vi "Structure Handler.vi"() -> ()   [LabVIEW 2010]
uses:
  <vilib>/Utility/miscctls.llb/LV3DPointTypeDef.ctl
  <vilib>/Analysis/Matrix/Datatypes/RealMatrix.ctl
  <vilib>/addons/database/_DB Variant To Data/Database Variant To Data.xnode
  <vilib>/addons/database/Connection.llb/DB Tools Open Connec (Path).vi
  <vilib>/addons/database/Connection.llb/Conn Execute.vi
  <vilib>/addons/database/Recordset.llb/Rec Fetch Recordset Data (R).vi
  <vilib>/addons/database/Recordset.llb/Rec Destroy - Connection.vi
  <vilib>/Analysis/_algsub.llb/Real Vector Norm.vi
  <vilib>/Utility/file.llb/Read From Spreadsheet File (string).vi
  <vilib>/Utility/file.llb/Write To Spreadsheet File (string).vi
  <vilib>/Analysis/baseanly.llb/Real Dot Product.vi
  <vilib>/addons/database/NI_Database_API.lvlib
  <vilib>/picture/3D Picture Control/NI_3D Picture Control.lvlib
  <vilib>/Analysis/NI_AALPro.lvlib
  <vilib>/Analysis/NI_AALBase.lvlib
  <vilib>/Analysis/Matrix/NI_Matrix.lvlib
panel:
  out "Last Structures":T1(array[cluster])
  out "x-y":u32[](array[numeric])
  out "Last Path":path caption="selected path"
  out "PickPoint":T2
  out "GB Subcrystal":T3={"Structure Name"="Batch6_3+111 Quasi-Bulk", "Lattice vector a"=[9.1641, 0.0, 0.0], "Lattice vector b"=[0.0, 7.93635, 0.0], "Lattice vector c"=[0.0, 0.0, 53.7091], "Atoms Array"=[{"Atom Name"="", "Positions (Direct)"=[[0.036896, 0.129554, 0.035254], [0.536896, 0.129554, 0.035254], [0.286896, 0.629554, 0.035254], [0.786896, 0.629554, 0.035254], [0.285415, 0.295133, 0.107673], [0.785415, 0.295133, 0.107673], [0.035415, 0.795133, 0.107673], [0.535415, 0.795133, 0.107673], [0.033615, 0.463308, 0.180101], [0.533615, 0.463308, 0.180101], [0.283615, 0.963308, 0.180101], [0.783615, 0.963308, 0.180101], [0.030844, 0.131453, 0.252535], [0.530844, 0.131453, 0.252535], [0.280844, 0.631453, 0.252535], [0.780844, 0.631453, 0.252535], [0.278379, 0.302058, 0.324923], [0.778379, 0.302058, 0.324923], [0.028379, 0.802058, 0.324923], [0.528379, 0.802058, 0.324923], [0.031198, 0.471844, 0.397363], [0.531198, 0.471844, 0.397363], [0.281198, 0.971844, 0.397363], [0.781198, 0.971844, 0.397363], [0.03247, 0.140643, 0.469814], [0.53247, 0.140643, 0.469814], [0.28247, 0.640643, 0.469814], [0.78247, 0.640643, 0.469814], [0.284308, 0.303948, 0.542263], [0.784308, 0.303948, 0.542263], [0.034308, 0.803948, 0.542263], [0.534308, 0.803948, 0.542263], [0.035944, 0.468219, 0.614701], [0.535944, 0.468219, 0.614701], [0.285944, 0.968219, 0.614701], [0.785944, 0.968219, 0.614701], [0.037813, 0.131858, 0.687216], [0.537813, 0.131858, 0.687216], [0.787813, 0.631858, 0.687216], [0.287813, 0.631858, 0.687216], [0.038238, 0.463759, 0.759817], [0.538238, 0.463759, 0.759817], [0.288238, 0.963758, 0.759817], [0.788238, 0.963758, 0.759817], [0.038639, 0.130134, 0.831025], [0.538639, 0.130134, 0.831025], [0.288639, 0.630134, 0.831025], [0.788639, 0.630134, 0.831025], [0.285712, 0.295024, 0.89873], [0.785712, 0.295024, 0.89873], [0.035712, 0.795024, 0.89873], [0.535712, 0.795024, 0.89873], [0.032596, 0.464879, 0.966384], [0.532596, 0.464879, 0.966384], [0.282596, 0.964879, 0.966384], [0.782596, 0.964879, 0.966384]], "Positions (Cartesian)"=[[0.33811863359999994, 1.0281858879, 1.8934606114], [4.9201686336, 1.0281858879, 1.8934606114], [2.6291436335999996, 4.9963608879, 1.8934606114], [7.2111936336, 4.9963608879, 1.8934606114], [2.6155716014999997, 2.34227878455, 5.7830199243000004], [7.197621601499999, 2.34227878455, 5.7830199243000004], [0.3245466015, 6.31045378455, 5.7830199243000004], [4.9065966014999995, 6.31045378455, 5.7830199243000004], [0.30805122149999997, 3.6769744458, 9.673062619100001], [4.890101221499999, 3.6769744458, 9.673062619100001], [2.5990762215, 7.6451494458, 9.673062619100001], [7.1811262215, 7.6451494458, 9.673062619100001], [0.2826575004, 1.04325701655, 13.5634275685], [4.8647075004, 1.04325701655, 13.5634275685], [2.5736825004, 5.011432016550001, 13.5634275685], [7.155732500399999, 5.011432016550001, 13.5634275685], [2.5510929938999998, 2.3972380083, 17.4513218993], [7.1331429939, 2.3972380083, 17.4513218993], [0.2600679939, 6.3654130083, 17.4513218993], [4.8421179939000005, 6.3654130083, 17.4513218993], [0.28590159179999997, 3.7447191294, 21.3420091033], [4.867951591799999, 3.7447191294, 21.3420091033], [2.5769265918, 7.7128941294, 21.3420091033], [7.158976591799999, 7.7128941294, 21.3420091033], [0.29755832699999996, 1.11619207305, 25.2332871074], [4.879608327, 1.11619207305, 25.2332871074], [2.588583327, 5.08436707305, 25.2332871074], [7.170633327, 5.08436707305, 25.2332871074], [2.6054269428, 2.4122377098, 29.124457693300002], [7.1874769428, 2.4122377098, 29.124457693300002], [0.31440194279999994, 6.3804127098, 29.124457693300002], [4.8964519428, 6.3804127098, 29.124457693300002], [0.32939441039999995, 3.71594986065, 33.0150374791], [4.9114444104, 3.71594986065, 33.0150374791], [2.6204194104, 7.684124860650001, 33.0150374791], [7.202469410399999, 7.684124860650001, 33.0150374791], [0.3465221133, 1.0464712383, 36.909752865600005], [4.9285721133, 1.0464712383, 36.909752865600005], [7.2195971133, 5.0146462383, 36.909752865600005], [2.6375471132999997, 5.0146462383, 36.909752865600005], [0.3504168558, 3.6805537396499997, 40.809087234699994], [4.9324668557999995, 3.6805537396499997, 40.809087234699994], [2.6414418557999997, 7.6487208033, 40.809087234699994], [7.2234918558, 7.6487208033, 40.809087234699994], [0.35409165989999997, 1.0327889709, 44.6336048275], [4.9361416599, 1.0327889709, 44.6336048275], [2.6451166599, 5.0009639709, 44.6336048275], [7.227166659899999, 5.0009639709, 44.6336048275], [2.6182933392, 2.3414137224, 48.269979443000004], [7.200343339199999, 2.3414137224, 48.269979443000004], [0.3272683392, 6.3095887224, 48.269979443000004], [4.9093183391999995, 6.3095887224, 48.269979443000004], [0.29871300359999997, 3.6894424516499997, 51.9036148944], [4.880763003599999, 3.6894424516499997, 51.9036148944], [2.5897380036, 7.65761745165, 51.9036148944], [7.171788003599999, 7.65761745165, 51.9036148944]]}, {"Atom Name"="", "Positions (Direct)"=[[0.286795, 0.296109, 0.054458], [0.786795, 0.296109, 0.054458], [0.036795, 0.796109, 0.054458], [0.536795, 0.796109, 0.054458], [0.035258, 0.462031, 0.126878], [0.535258, 0.462031, 0.126878], [0.285258, 0.962031, 0.126878], [0.785258, 0.962031, 0.126878], [0.033445, 0.130094, 0.199309], [0.533445, 0.130094, 0.199309], [0.283445, 0.630094, 0.199309], [0.783445, 0.630094, 0.199309], [0.280766, 0.298203, 0.27171], [0.780766, 0.298203, 0.27171], [0.030766, 0.798203, 0.27171], [0.530766, 0.798203, 0.27171], [0.028505, 0.468822, 0.344121], [0.528505, 0.468822, 0.344121], [0.278505, 0.968822, 0.344121], [0.778505, 0.968822, 0.344121], [0.03126, 0.138635, 0.416572], [0.53126, 0.138635, 0.416572], [0.28126, 0.638635, 0.416572], [0.78126, 0.638635, 0.416572], [0.282556, 0.307128, 0.489026], [0.782556, 0.307128, 0.489026], [0.032556, 0.807128, 0.489026], [0.532556, 0.807128, 0.489026], [0.034374, 0.470438, 0.56147], [0.534374, 0.470438, 0.56147], [0.284374, 0.970438, 0.56147], [0.784374, 0.970438, 0.56147], [0.035964, 0.134698, 0.633895], [0.535964, 0.134698, 0.633895], [0.285964, 0.634698, 0.633895], [0.785964, 0.634698, 0.633895], [0.037794, 0.465111, 0.706493], [0.537794, 0.465111, 0.706493], [0.787794, 0.965111, 0.706493], [0.287794, 0.965111, 0.706493], [0.038181, 0.130274, 0.779081], [0.538181, 0.130274, 0.779081], [0.288181, 0.630273, 0.779081], [0.788181, 0.630273, 0.779081], [0.288548, 0.296604, 0.847022], [0.788548, 0.296604, 0.847022], [0.038548, 0.796604, 0.847022], [0.538548, 0.796604, 0.847022], [0.035661, 0.461866, 0.914714], [0.535661, 0.461866, 0.914714], [0.285661, 0.961866, 0.914714], [0.785661, 0.961866, 0.914714], [0.032517, 0.131341, 0.982331], [0.532517, 0.131341, 0.982331], [0.282517, 0.631341, 0.982331], [0.782517, 0.631341, 0.982331]], "Positions (Cartesian)"=[[2.6282180595, 2.35002466215, 2.9248901678], [7.2102680595, 2.35002466215, 2.9248901678], [0.3371930595, 6.31819966215, 2.9248901678], [4.9192430595, 6.31819966215, 2.9248901678], [0.32310783779999996, 3.66683972685, 6.814503189799999], [4.9051578378, 3.66683972685, 6.814503189799999], [2.6141328378, 7.63501472685, 6.814503189799999], [7.1961828377999995, 7.63501472685, 6.814503189799999], [0.3064933245, 1.0324715168999998, 10.704707011899998], [4.8885433245, 1.0324715168999998, 10.704707011899998], [2.5975183244999998, 5.000646516900001, 10.704707011899998], [7.179568324499999, 5.000646516900001, 10.704707011899998], [2.5729677006, 2.36664337905, 14.593299561], [7.155017700599999, 2.36664337905, 14.593299561], [0.2819427006, 6.33481837905, 14.593299561], [4.863992700599999, 6.33481837905, 14.593299561], [0.2612226705, 3.7207354797, 18.4824292011], [4.843272670499999, 3.7207354797, 18.4824292011], [2.5522476705, 7.6889104797, 18.4824292011], [7.1342976705, 7.6889104797, 18.4824292011], [0.286469766, 1.1002558822500002, 22.3737072052], [4.8685197659999995, 1.1002558822500002, 22.3737072052], [2.577494766, 5.0684308822499995, 22.3737072052], [7.159544765999999, 5.0684308822499995, 22.3737072052], [2.5893714396, 2.4374753028000002, 26.2651463366], [7.1714214396, 2.4374753028000002, 26.2651463366], [0.2983464396, 6.4056503028, 26.2651463366], [4.8803964396, 6.4056503028, 26.2651463366], [0.3150067734, 3.7335606213, 30.156048377], [4.8970567734, 3.7335606213, 30.156048377], [2.6060317734, 7.7017356213, 30.156048377], [7.1880817733999995, 7.7017356213, 30.156048377], [0.3295776924, 1.0690104723, 34.045929944499996], [4.9116276924, 1.0690104723, 34.045929944499996], [2.6206026924, 5.0371854723, 34.045929944499996], [7.202652692399999, 5.0371854723, 34.045929944499996], [0.3463479954, 3.69128368485, 37.9451031863], [4.928397995399999, 3.69128368485, 37.9451031863], [7.2194229953999995, 7.659458684850001, 37.9451031863], [2.6373729954, 7.659458684850001, 37.9451031863], [0.34989450209999995, 1.0339000599000001, 41.843739337100004], [4.9319445020999995, 1.0339000599000001, 41.843739337100004], [2.6409195021, 5.00206712355, 41.843739337100004], [7.2229695021, 5.00206712355, 41.843739337100004], [2.6442827268, 2.3539531553999997, 45.4927893002], [7.2263327268, 2.3539531553999997, 45.4927893002], [0.35325772679999995, 6.3221281554, 45.4927893002], [4.9353077268, 6.3221281554, 45.4927893002], [0.3268009701, 3.6655302291, 49.1284656974], [4.9088509701000005, 3.6655302291, 49.1284656974], [2.6178259700999997, 7.6337052291, 49.1284656974], [7.1998759701, 7.6337052291, 49.1284656974], [0.29798903969999996, 1.04236814535, 52.760113912099996], [4.8800390397, 1.04236814535, 52.760113912099996], [2.5890140397, 5.010543145350001, 52.760113912099996], [7.1710640397, 5.010543145350001, 52.760113912099996]]}], "# of atoms"=112}
  out "Structure ID":string="Batch6_3+111 Quasi-Bulk"
  out "Exists?":bool
  in  "Structure Name":string="1_A13B_utwin"
  in  "Main Tabs":T4(tab)=enum."Structure Analysis"
  in  "Upload Download":enum32{"Download", "Upload", "Grow your own"}(tab)
  in  "Apply Filter":bool
  in  "Database Entries":i32(listbox)
  in  "Query Filter":T5={"Sample Check box"=FALSE, "Sample Comparison Type"="Contains", "Sample Name"="", "Logical Sample-Lot "="OR", "LotID Checkbox"=FALSE, "Lot Comparison Type"="Is exactly", "LotID Name"="", "Logical Lot-Date"="OR", "Date Checkbox"=FALSE, "Start Date"=timestamp(3375812149.928578 s since 1904-01-01), "End Date"=timestamp(3375812149.928578 s since 1904-01-01), "1st search column name"="Structure_Name", "2nd search column name"="Folder"} {"Start Date" format="%<%X\n%x>T"; "End Date" format="%<%X\n%x>T"}
  in  "Database UDL":path=path "D:/Ab-initio/VASP Calcs/VASP DB.udl"
  in  "Structure Cluster":T6={"Defect Dimention"=2, "Defect Type"="Grain Boundary", "Intrinsic or Extrinsic"="Intrinsic", "Comments"="0"}
  in  "Send Structure to DB":bool
  in  "Save to File":bool
  in  "Structure Manip Options":T7(tab)
  in  "Add Crop Rotate Tabs":T8(tab)
  in  "Padding Options":i32(listbox)
  in  "Where to pad?":enum32{"Pad on Left", "Pad on Right"}(radio)
  in  "Add Bulk":bool
  in  "Supercell Draw Box X":cluster{dbl, dbl}(slide) scale=-1.0..30.0
  in  "Supercell Draw Box Y":cluster{dbl, dbl}(slide) scale=0.0..30.0
  in  "Supercell Draw Box Z":cluster{dbl, dbl}(slide) scale=-1.0..99.0
  in  "b lattice factor":i16=1 caption="b" min=1 max=1000 step=1
  in  "c lattice factor":i16=1 caption="c" min=1 max=1000 step=1
  in  "a lattice factor":i16=1 caption="a" min=1 max=1000 step=1
  in  "Prickle Distance (A)":dbl(slide) scale=0.0..6.0
  in  "Suggest Supercell Draw Box":bool
  in  "Crop Range":cluster{dbl, dbl}(slide)={0.0, 46.0} scale=-1.0..35.16419204615208
  in  "Cropping Index":enum16{"X", "Y", "Z"}(ring)=enum."Z"
  in  "Remove Close Atoms":bool
  in  "Minimally Allowable Distance (A)":dbl=1.5
  out "# of Atoms Removed":i32
  in  "Lock c":bool
  in  "Lock b":bool
  in  "New c Axis":dbl[](array[numeric])=[1.0, 0.0, 0.0]
  in  "New b Axis":dbl[](array[numeric])=[1.0, 0.0, 0.0]
  in  "New a Axis":dbl[](array[numeric])=[1.0, 0.0, 0.0]
  in  "Rotation":dbl(slide) scale=0.0..360.0
  in  "Rotation Axis":dbl[](array[numeric])=[1.0, 0.0, 0.0]
  in  "Matrix Transform":T9=[[1.0, 0.0, 0.0], [0.0, 6.123233995736766e-17, 1.0], [0.0, -1.0, 6.123233995736766e-17]]
  in  "Lock a":bool
  in  "Translation Vector (Cartesian)":dbl[](array[numeric])=[9.1641, 0.0, 0.0]
  in  "Map to [0,1)":bool
  in  "0D Defects tab":enum32{"Single Defects", "Defect Pairs"}(tab)
  in  "Highlight Color":u32(colorbox)
  in  "Replacement Atom":string(combo) caption="New Atom"
  in  "Replace Atom":bool
  in  "Add Interstitial":bool
  in  "Highlight During Selection?":bool
  in  "Atom List":i32[](listbox)
  in  "Make Vacancy":bool
  in  "Defect 1 Atom Index":i32
  in  "Minimum Distance":dbl
  in  "Maximum Distnce":dbl=8.0
  in  "Make defect pair":bool
  in  "Defect 1":cluster{"Species":string, "Defect Type":string}={"Species"="Te", "Defect Type"="Substitutional"}
  in  "Defect 2":cluster{"Species":string, "Defect Type":string}={"Species"="Te", "Defect Type"="Interstitial, Tetra, Unlike atoms"}
  in  "Rotation Axis Intersection":dbl[](array[numeric])=[1.0, 0.0, 0.0]
  in  "Twist Angle":dbl(slide) scale=0.0..120.0
  in  "Tilt Angle":dbl(slide) scale=0.0..180.0
  in  "Show New Grain":bool
  in  "Base Atom":i32
  in  "GB Draw Box X":cluster{dbl, dbl}(slide) scale=-1.0..10.0
  in  "GB Draw Box Y":cluster{dbl, dbl}(slide) scale=-1.0..60.0
  in  "GB Draw Box Z":cluster{dbl, dbl}(slide) scale=-5.0..50.0
  in  "Suggest Draw Box":bool
  in  "Predict Best Strain":bool
  in  "Additional Strain/twin (A)":dbl(slide) scale=0.0..1.0
  in  "Periodicity":i32[](array[numeric])=[3, 3]
  out "# of extra cells needed for cubic":i32
  in  "Current Atomic Structure":T3={"Structure Name"="Batch6_3+111 Quasi-Bulk", "Lattice vector a"=[9.1641, 0.0, 0.0], "Lattice vector b"=[0.0, 7.93635, 0.0], "Lattice vector c"=[0.0, 0.0, 53.7091], "Atoms Array"=[{"Atom Name"="", "Positions (Direct)"=[[0.036896, 0.129554, 0.035254], [0.536896, 0.129554, 0.035254], [0.286896, 0.629554, 0.035254], [0.786896, 0.629554, 0.035254], [0.285415, 0.295133, 0.107673], [0.785415, 0.295133, 0.107673], [0.035415, 0.795133, 0.107673], [0.535415, 0.795133, 0.107673], [0.033615, 0.463308, 0.180101], [0.533615, 0.463308, 0.180101], [0.283615, 0.963308, 0.180101], [0.783615, 0.963308, 0.180101], [0.030844, 0.131453, 0.252535], [0.530844, 0.131453, 0.252535], [0.280844, 0.631453, 0.252535], [0.780844, 0.631453, 0.252535], [0.278379, 0.302058, 0.324923], [0.778379, 0.302058, 0.324923], [0.028379, 0.802058, 0.324923], [0.528379, 0.802058, 0.324923], [0.031198, 0.471844, 0.397363], [0.531198, 0.471844, 0.397363], [0.281198, 0.971844, 0.397363], [0.781198, 0.971844, 0.397363], [0.03247, 0.140643, 0.469814], [0.53247, 0.140643, 0.469814], [0.28247, 0.640643, 0.469814], [0.78247, 0.640643, 0.469814], [0.284308, 0.303948, 0.542263], [0.784308, 0.303948, 0.542263], [0.034308, 0.803948, 0.542263], [0.534308, 0.803948, 0.542263], [0.035944, 0.468219, 0.614701], [0.535944, 0.468219, 0.614701], [0.285944, 0.968219, 0.614701], [0.785944, 0.968219, 0.614701], [0.037813, 0.131858, 0.687216], [0.537813, 0.131858, 0.687216], [0.787813, 0.631858, 0.687216], [0.287813, 0.631858, 0.687216], [0.038238, 0.463759, 0.759817], [0.538238, 0.463759, 0.759817], [0.288238, 0.963758, 0.759817], [0.788238, 0.963758, 0.759817], [0.038639, 0.130134, 0.831025], [0.538639, 0.130134, 0.831025], [0.288639, 0.630134, 0.831025], [0.788639, 0.630134, 0.831025], [0.285712, 0.295024, 0.89873], [0.785712, 0.295024, 0.89873], [0.035712, 0.795024, 0.89873], [0.535712, 0.795024, 0.89873], [0.032596, 0.464879, 0.966384], [0.532596, 0.464879, 0.966384], [0.282596, 0.964879, 0.966384], [0.782596, 0.964879, 0.966384]], "Positions (Cartesian)"=[[0.33811863359999994, 1.0281858879, 1.8934606114], [4.9201686336, 1.0281858879, 1.8934606114], [2.6291436335999996, 4.9963608879, 1.8934606114], [7.2111936336, 4.9963608879, 1.8934606114], [2.6155716014999997, 2.34227878455, 5.7830199243000004], [7.197621601499999, 2.34227878455, 5.7830199243000004], [0.3245466015, 6.31045378455, 5.7830199243000004], [4.9065966014999995, 6.31045378455, 5.7830199243000004], [0.30805122149999997, 3.6769744458, 9.673062619100001], [4.890101221499999, 3.6769744458, 9.673062619100001], [2.5990762215, 7.6451494458, 9.673062619100001], [7.1811262215, 7.6451494458, 9.673062619100001], [0.2826575004, 1.04325701655, 13.5634275685], [4.8647075004, 1.04325701655, 13.5634275685], [2.5736825004, 5.011432016550001, 13.5634275685], [7.155732500399999, 5.011432016550001, 13.5634275685], [2.5510929938999998, 2.3972380083, 17.4513218993], [7.1331429939, 2.3972380083, 17.4513218993], [0.2600679939, 6.3654130083, 17.4513218993], [4.8421179939000005, 6.3654130083, 17.4513218993], [0.28590159179999997, 3.7447191294, 21.3420091033], [4.867951591799999, 3.7447191294, 21.3420091033], [2.5769265918, 7.7128941294, 21.3420091033], [7.158976591799999, 7.7128941294, 21.3420091033], [0.29755832699999996, 1.11619207305, 25.2332871074], [4.879608327, 1.11619207305, 25.2332871074], [2.588583327, 5.08436707305, 25.2332871074], [7.170633327, 5.08436707305, 25.2332871074], [2.6054269428, 2.4122377098, 29.124457693300002], [7.1874769428, 2.4122377098, 29.124457693300002], [0.31440194279999994, 6.3804127098, 29.124457693300002], [4.8964519428, 6.3804127098, 29.124457693300002], [0.32939441039999995, 3.71594986065, 33.0150374791], [4.9114444104, 3.71594986065, 33.0150374791], [2.6204194104, 7.684124860650001, 33.0150374791], [7.202469410399999, 7.684124860650001, 33.0150374791], [0.3465221133, 1.0464712383, 36.909752865600005], [4.9285721133, 1.0464712383, 36.909752865600005], [7.2195971133, 5.0146462383, 36.909752865600005], [2.6375471132999997, 5.0146462383, 36.909752865600005], [0.3504168558, 3.6805537396499997, 40.809087234699994], [4.9324668557999995, 3.6805537396499997, 40.809087234699994], [2.6414418557999997, 7.6487208033, 40.809087234699994], [7.2234918558, 7.6487208033, 40.809087234699994], [0.35409165989999997, 1.0327889709, 44.6336048275], [4.9361416599, 1.0327889709, 44.6336048275], [2.6451166599, 5.0009639709, 44.6336048275], [7.227166659899999, 5.0009639709, 44.6336048275], [2.6182933392, 2.3414137224, 48.269979443000004], [7.200343339199999, 2.3414137224, 48.269979443000004], [0.3272683392, 6.3095887224, 48.269979443000004], [4.9093183391999995, 6.3095887224, 48.269979443000004], [0.29871300359999997, 3.6894424516499997, 51.9036148944], [4.880763003599999, 3.6894424516499997, 51.9036148944], [2.5897380036, 7.65761745165, 51.9036148944], [7.171788003599999, 7.65761745165, 51.9036148944]]}, {"Atom Name"="", "Positions (Direct)"=[[0.286795, 0.296109, 0.054458], [0.786795, 0.296109, 0.054458], [0.036795, 0.796109, 0.054458], [0.536795, 0.796109, 0.054458], [0.035258, 0.462031, 0.126878], [0.535258, 0.462031, 0.126878], [0.285258, 0.962031, 0.126878], [0.785258, 0.962031, 0.126878], [0.033445, 0.130094, 0.199309], [0.533445, 0.130094, 0.199309], [0.283445, 0.630094, 0.199309], [0.783445, 0.630094, 0.199309], [0.280766, 0.298203, 0.27171], [0.780766, 0.298203, 0.27171], [0.030766, 0.798203, 0.27171], [0.530766, 0.798203, 0.27171], [0.028505, 0.468822, 0.344121], [0.528505, 0.468822, 0.344121], [0.278505, 0.968822, 0.344121], [0.778505, 0.968822, 0.344121], [0.03126, 0.138635, 0.416572], [0.53126, 0.138635, 0.416572], [0.28126, 0.638635, 0.416572], [0.78126, 0.638635, 0.416572], [0.282556, 0.307128, 0.489026], [0.782556, 0.307128, 0.489026], [0.032556, 0.807128, 0.489026], [0.532556, 0.807128, 0.489026], [0.034374, 0.470438, 0.56147], [0.534374, 0.470438, 0.56147], [0.284374, 0.970438, 0.56147], [0.784374, 0.970438, 0.56147], [0.035964, 0.134698, 0.633895], [0.535964, 0.134698, 0.633895], [0.285964, 0.634698, 0.633895], [0.785964, 0.634698, 0.633895], [0.037794, 0.465111, 0.706493], [0.537794, 0.465111, 0.706493], [0.787794, 0.965111, 0.706493], [0.287794, 0.965111, 0.706493], [0.038181, 0.130274, 0.779081], [0.538181, 0.130274, 0.779081], [0.288181, 0.630273, 0.779081], [0.788181, 0.630273, 0.779081], [0.288548, 0.296604, 0.847022], [0.788548, 0.296604, 0.847022], [0.038548, 0.796604, 0.847022], [0.538548, 0.796604, 0.847022], [0.035661, 0.461866, 0.914714], [0.535661, 0.461866, 0.914714], [0.285661, 0.961866, 0.914714], [0.785661, 0.961866, 0.914714], [0.032517, 0.131341, 0.982331], [0.532517, 0.131341, 0.982331], [0.282517, 0.631341, 0.982331], [0.782517, 0.631341, 0.982331]], "Positions (Cartesian)"=[[2.6282180595, 2.35002466215, 2.9248901678], [7.2102680595, 2.35002466215, 2.9248901678], [0.3371930595, 6.31819966215, 2.9248901678], [4.9192430595, 6.31819966215, 2.9248901678], [0.32310783779999996, 3.66683972685, 6.814503189799999], [4.9051578378, 3.66683972685, 6.814503189799999], [2.6141328378, 7.63501472685, 6.814503189799999], [7.1961828377999995, 7.63501472685, 6.814503189799999], [0.3064933245, 1.0324715168999998, 10.704707011899998], [4.8885433245, 1.0324715168999998, 10.704707011899998], [2.5975183244999998, 5.000646516900001, 10.704707011899998], [7.179568324499999, 5.000646516900001, 10.704707011899998], [2.5729677006, 2.36664337905, 14.593299561], [7.155017700599999, 2.36664337905, 14.593299561], [0.2819427006, 6.33481837905, 14.593299561], [4.863992700599999, 6.33481837905, 14.593299561], [0.2612226705, 3.7207354797, 18.4824292011], [4.843272670499999, 3.7207354797, 18.4824292011], [2.5522476705, 7.6889104797, 18.4824292011], [7.1342976705, 7.6889104797, 18.4824292011], [0.286469766, 1.1002558822500002, 22.3737072052], [4.8685197659999995, 1.1002558822500002, 22.3737072052], [2.577494766, 5.0684308822499995, 22.3737072052], [7.159544765999999, 5.0684308822499995, 22.3737072052], [2.5893714396, 2.4374753028000002, 26.2651463366], [7.1714214396, 2.4374753028000002, 26.2651463366], [0.2983464396, 6.4056503028, 26.2651463366], [4.8803964396, 6.4056503028, 26.2651463366], [0.3150067734, 3.7335606213, 30.156048377], [4.8970567734, 3.7335606213, 30.156048377], [2.6060317734, 7.7017356213, 30.156048377], [7.1880817733999995, 7.7017356213, 30.156048377], [0.3295776924, 1.0690104723, 34.045929944499996], [4.9116276924, 1.0690104723, 34.045929944499996], [2.6206026924, 5.0371854723, 34.045929944499996], [7.202652692399999, 5.0371854723, 34.045929944499996], [0.3463479954, 3.69128368485, 37.9451031863], [4.928397995399999, 3.69128368485, 37.9451031863], [7.2194229953999995, 7.659458684850001, 37.9451031863], [2.6373729954, 7.659458684850001, 37.9451031863], [0.34989450209999995, 1.0339000599000001, 41.843739337100004], [4.9319445020999995, 1.0339000599000001, 41.843739337100004], [2.6409195021, 5.00206712355, 41.843739337100004], [7.2229695021, 5.00206712355, 41.843739337100004], [2.6442827268, 2.3539531553999997, 45.4927893002], [7.2263327268, 2.3539531553999997, 45.4927893002], [0.35325772679999995, 6.3221281554, 45.4927893002], [4.9353077268, 6.3221281554, 45.4927893002], [0.3268009701, 3.6655302291, 49.1284656974], [4.9088509701000005, 3.6655302291, 49.1284656974], [2.6178259700999997, 7.6337052291, 49.1284656974], [7.1998759701, 7.6337052291, 49.1284656974], [0.29798903969999996, 1.04236814535, 52.760113912099996], [4.8800390397, 1.04236814535, 52.760113912099996], [2.5890140397, 5.010543145350001, 52.760113912099996], [7.1710640397, 5.010543145350001, 52.760113912099996]]}], "# of atoms"=112}
  in  "Accept These Changes":bool
  in  "Undo Last":bool
  in  "Axis":i32(slide) scale=0.0..2.0
  in  "Max Bond Length":dbl
  out "System XY Graph":cluster{dbl, dbl}[](graph)
  in  "VASP Tab":T10(tab)
  in  "Wiggle one atom by 0.1%":bool=TRUE
  in  "Add to final POTCAR":bool
  in  "Available POTCARs":i32(listbox)
  in  "POTCAR Array":string[](array[combo])=["PAW_PBE Cd 06Sep2000", "PAW_PBE Te 08Apr2002"]
  in  "Write # comment":bool
  in  "INCAR File":string
  in  "INCAR Defaults":i32(listbox)
  in  "Command":string(combo)
  in  "Value":string(combo)
  out "Description":string
  in  "K-Points Tab":enum32{"Automatic", "Manual"}(tab)
  in  "Auto Type":T11(radio)
  in  "|G| Factor":dbl=30.0
  in  "Symmetry":enum32{"High-Symmetry", "L-G-X", "Manual Mesh"}(radio)
  in  "# Points between":i32
  in  "Manual Type":enum32{"Reciprocal", "Cartesian"}(radio)
  in  "K-point Mesh":T12(array[cluster])
  out "K-Points File":string="Automatic Mesh\n-1\nGamma Centered Monkhurst-Pack\n  4 4 1\n"
  in  "Values":string[](array[string])=["Structure ID", "Structure Name"]
  in  "Headers":string[](array[string])=["Structure ID", "Structure Name"]
  in  "Email?":T13={"Email at Beginning?"=FALSE, "Email at End?"=FALSE, "Email when aborted?"=TRUE}
  in  "Expected Walltime":dbl=172800.0 format="%<%H:%M:%S>t"
  in  "Load VTST for NEB?":bool
  in  "Nodes and Processors":T14={"Number of Nodes"=4, "Processors per node"=8}
  in  "CNM Contract Name":string(combo)="cnm40004"
  in  "VASPify":bool
  in  "VASPIFY Folder Name":string="1_A13B_utwin"
  in  "GULP":bool
  in  "Title":string
  in  "Relaxation Type":string(combo)="conv opti"
  in  "Lattice Vectors":T15={"Lattice Vector Type"=enum."Vectors", "DoF to Allow Relaxation?"=[1, 1, 1, 1, 1, 1]}
  in  "Potentials":T16={"Potential Used"="sw2", "Potential Details"=[{"Atom 1"="Cd core", "Atom 2"="Te core", "Parameters"=[7.261088, 2.51, 23.9020768], "Range Min (A)"=0.0, "Range Max (A)"=4.518}, {"Atom 1"="Cd core", "Atom 2"="Cd core", "Parameters"=[5.327778, 2.51, 34.9560927], "Range Min (A)"=0.0, "Range Max (A)"=4.518}, {"Atom 1"="Te core", "Atom 2"="Te core", "Parameters"=[8.385745, 2.51, 26.4780396], "Range Min (A)"=0.0, "Range Max (A)"=4.518}]}
  out "Base Object":refnum<vi>
  in  "Base 111 Structures":T1(array[cluster])=[{"Structure Name"="111 A3 (vnl down) bulk, Cd Terminated.cif", "Lattice vector a"=[4.67354, 0.0, 0.0], "Lattice vector b"=[0.0, 8.0948, 0.0], "Lattice vector c"=[0.0, 0.0, 11.4478], "Atoms Array"=[{"Atom Name"="Cd", "Positions (Direct)"=[[0.0, 0.333334, 0.083333], [0.500001, 0.833335, 0.083333], [0.500001, 0.166667, 0.416667], [0.0, 0.666668, 0.416667], [0.0, 0.0, 0.75], [0.500001, 0.500001, 0.75]], "Positions (Cartesian)"=[[0.0, 2.6982720632, 0.9539795174000001], [2.3367746735400003, 6.745680158, 0.9539795174000001], [2.3367746735400003, 1.3491360316, 4.769920482600001], [0.0, 5.3965441264, 4.769920482600001], [0.0, 0.0, 8.58585], [2.3367746735400003, 4.0474080948, 8.58585]]}, {"Atom Name"="Te", "Positions (Direct)"=[[0.0, 0.0, 0.0], [0.500001, 0.500001, 0.0], [0.0, 0.333334, 0.333334], [0.500001, 0.833335, 0.333334], [0.500001, 0.166667, 0.666667], [0.0, 0.666668, 0.666667]], "Positions (Cartesian)"=[[0.0, 0.0, 0.0], [2.3367746735400003, 4.0474080948, 0.0], [0.0, 2.6982720632, 3.8159409652000007], [2.3367746735400003, 6.745680158, 3.8159409652000007], [2.3367746735400003, 1.3491360316, 7.631870482600001], [0.0, 5.3965441264, 7.631870482600001]]}], "# of atoms"=12}, {"Structure Name"="111 A3 (vnl down) bulk, Te Terminated.cif", "Lattice vector a"=[4.67354, 0.0, 0.0], "Lattice vector b"=[0.0, 8.0948, 0.0], "Lattice vector c"=[0.0, 0.0, 11.4478], "Atoms Array"=[{"Atom Name"="Cd", "Positions (Direct)"=[[0.0, 0.0, 0.0], [0.500001, 0.500001, 0.0], [0.0, 0.333334, 0.333334], [0.500001, 0.833335, 0.333334], [0.500001, 0.166667, 0.666667], [0.0, 0.666668, 0.666667]], "Positions (Cartesian)"=[[0.0, 0.0, 0.0], [2.3367746735400003, 4.0474080948, 0.0], [0.0, 2.6982720632, 3.8159409652000007], [2.3367746735400003, 6.745680158, 3.8159409652000007], [2.3367746735400003, 1.3491360316, 7.631870482600001], [0.0, 5.3965441264, 7.631870482600001]]}, {"Atom Name"="Te", "Positions (Direct)"=[[0.0, 0.333334, 0.083333], [0.500001, 0.833335, 0.083333], [0.500001, 0.166667, 0.416667], [0.0, 0.666668, 0.416667], [0.0, 0.0, 0.75], [0.500001, 0.500001, 0.75]], "Positions (Cartesian)"=[[0.0, 2.6982720632, 0.9539795174000001], [2.3367746735400003, 6.745680158, 0.9539795174000001], [2.3367746735400003, 1.3491360316, 4.769920482600001], [0.0, 5.3965441264, 4.769920482600001], [0.0, 0.0, 8.58585], [2.3367746735400003, 4.0474080948, 8.58585]]}], "# of atoms"=12}, {"Structure Name"="111 A3 (vnl up) bulk, Cd Terminated.cif", "Lattice vector a"=[4.67354, 0.0, 0.0], "Lattice vector b"=[0.0, 8.0948, 0.0], "Lattice vector c"=[0.0, 0.0, 11.4478], "Atoms Array"=[{"Atom Name"="Cd", "Positions (Direct)"=[[0.0, 0.333334, 0.666667], [0.500001, 0.833335, 0.666667], [0.500001, 0.166667, 0.333333], [0.0, 0.666668, 0.333333], [0.0, 0.0, 0.0], [0.500001, 0.500001, 0.0]], "Positions (Cartesian)"=[[0.0, 2.6982720632, 7.631870482600001], [2.3367746735400003, 6.745680158, 7.631870482600001], [2.3367746735400003, 1.3491360316, 3.8159295174000003], [0.0, 5.3965441264, 3.8159295174000003], [0.0, 0.0, 0.0], [2.3367746735400003, 4.0474080948, 0.0]]}, {"Atom Name"="Te", "Positions (Direct)"=[[0.0, 0.0, 0.75], [0.500001, 0.500001, 0.75], [0.0, 0.333334, 0.416666], [0.500001, 0.833335, 0.416666], [0.500001, 0.166667, 0.083333], [0.0, 0.666668, 0.083333]], "Positions (Cartesian)"=[[0.0, 0.0, 8.58585], [2.3367746735400003, 4.0474080948, 8.58585], [0.0, 2.6982720632, 4.7699090348], [2.3367746735400003, 6.745680158, 4.7699090348], [2.3367746735400003, 1.3491360316, 0.9539795174000001], [0.0, 5.3965441264, 0.9539795174000001]]}], "# of atoms"=12}, {"Structure Name"="111 A3 (vnl up) bulk, Te Terminated.cif", "Lattice vector a"=[4.67354, 0.0, 0.0], "Lattice vector b"=[0.0, 8.0948, 0.0], "Lattice vector c"=[0.0, 0.0, 11.4478], "Atoms Array"=[{"Atom Name"="Cd", "Positions (Direct)"=[[0.0, 0.0, 0.75], [0.500001, 0.500001, 0.75], [0.0, 0.333334, 0.416666], [0.500001, 0.833335, 0.416666], [0.500001, 0.166667, 0.083333], [0.0, 0.666668, 0.083333]], "Positions (Cartesian)"=[[0.0, 0.0, 8.58585], [2.3367746735400003, 4.0474080948, 8.58585], [0.0, 2.6982720632, 4.7699090348], [2.3367746735400003, 6.745680158, 4.7699090348], [2.3367746735400003, 1.3491360316, 0.9539795174000001], [0.0, 5.3965441264, 0.9539795174000001]]}, {"Atom Name"="Te", "Positions (Direct)"=[[0.0, 0.333334, 0.666667], [0.500001, 0.833335, 0.666667], [0.500001, 0.166667, 0.333333], [0.0, 0.666668, 0.333333], [0.0, 0.0, 0.0], [0.500001, 0.500001, 0.0]], "Positions (Cartesian)"=[[0.0, 2.6982720632, 7.631870482600001], [2.3367746735400003, 6.745680158, 7.631870482600001], [2.3367746735400003, 1.3491360316, 3.8159295174000003], [0.0, 5.3965441264, 3.8159295174000003], [0.0, 0.0, 0.0], [2.3367746735400003, 4.0474080948, 0.0]]}], "# of atoms"=12}, {"Structure Name"="111 A1B1 Twin Column (vnl up, down), Te Terminated.cif", "Lattice vector a"=[4.67354, 0.0, 0.0], "Lattice vector b"=[0.0, 8.0948, 0.0], "Lattice vector c"=[0.0, 0.0, 7.63187], "Atoms Array"=[{"Atom Name"="Cd", "Positions (Direct)"=[[0.0, 0.0, 0.0], [0.500001, 0.500001, 0.0], [0.500001, 0.166667, 0.5], [1.84889e-32, 0.666668, 0.5]], "Positions (Cartesian)"=[[0.0, 0.0, 0.0], [2.3367746735400003, 4.0474080948, 0.0], [2.3367746735400003, 1.3491360316, 3.815935], [8.640861370600001e-32, 5.3965441264, 3.815935]]}, {"Atom Name"="Te", "Positions (Direct)"=[[0.500001, 0.166667, 0.11033], [1.38667e-32, 0.666668, 0.11033], [-1.2326e-32, -1.2326e-32, 0.625], [0.500001, 0.500001, 0.625]], "Positions (Cartesian)"=[[2.3367746735400003, 1.3491360316, 0.8420242171], [6.4806577118e-32, 5.3965441264, 0.8420242171], [-5.760605403999999e-32, -9.977650479999997e-32, 4.76991875], [2.3367746735400003, 4.0474080948, 4.76991875]]}], "# of atoms"=8}]
  out "POTCAR File":string=" PAW_PBE Cd 06Sep2000\n 12.0000000000000000\n parameters from PSCTR are:\n   VRHFIN =Cd : s2 d10\n   LEXCH  = PE\n   EATOM  =  1293.2795 eV,   95.0534 Ry\n\n   TITEL  = PAW_PBE Cd 06Sep2000\n   LULTRA =        F    use ultrasoft PP ?\n   IUNSCR =        1    unscreen: 0-lin 1-nonlin 2-no\n   RPACOR =    2.000    partial core radius\n   POMASS =  112.411; ZVAL   =   12.000    mass and valenz\n   RCORE  =    2.300    outmost cutoff radius\n   RWIGS  =    2.980; RWIGS  =    1.577    wigner-seitz radius (au A)\n   ENMAX  =  274.342; ENMIN  =  205.757 eV\n   RCLOC  =    2.054    cutoff for local pot\n   LCOR   =        T    correct aug charges\n   LPAW   =        T    paw PP\n   EAUG   =  456.106\n   DEXC   =    -.021\n   RMAX   =    2.784    core radius for proj-oper\n   RAUG   =    1.300    factor for augmentation sphere\n   RDEP   =    2.450    radius for radial grids\n   QCUT   =   -4.490; QGAM   =    8.981    optimization parameters\n \n   Description\n     l     E      TYP  RCUT    TYP  RCUT\n     2   .000     23  2.300\n     2   .000     23  2.300\n     0   .000     23  2.300\n     0   .000     23  2.300\n     1  -.200     23  2.300\n     1   .000     23  2.300\n     3   .000      7   .000\n   Error from kinetic energy argument (eV)\n   NDATA  =      100\n   STEP   =   20.000   1.050\n  208.      207.      206.      203.      202.      200.      197.      196.\n  192.      189.      187.      184.      180.      176.      171.      167.\n  162.      158.      153.      145.      140.      134.      126.      121.\n  116.      108.      99.5      94.3      86.5      79.0      71.8      64.9\n  58.3      52.0      46.2      40.8      34.2      29.7      24.4      20.8\n  16.7      13.2      10.2      7.82      5.86      4.31      3.10      1.98\n  1.34      .796      .452      .281      .156      .959E-01  .691E-01  .641E-01\n  .637E-01  .620E-01  .562E-01  .469E-01  .360E-01  .258E-01  .175E-01  .110E-01\n  .798E-02  .656E-02  .628E-02  .621E-02  .576E-02  .494E-02  .373E-02  .260E-02\n  .179E-02  .138E-02  .124E-02  .122E-02  .116E-02  .989E-03  .732E-03  .527E-03\n  .392E-03  .349E-03  .342E-03  .317E-03  .256E-03  .187E-03  .141E-03  .123E-03\n  .120E-03  .109E-03  .840E-04  .629E-04  .520E-04  .502E-04  .456E-04  .358E-04\n  .268E-04  .240E-04  .229E-04  .193E-04\nEND of PSCTR-controll parameters\n local part\n 81.2582175088937078\n   .18547413E+03   .18542997E+03   .18529762E+03   .18507728E+03   .18476934E+03\n   .18437431E+03   .18389284E+03   .18332575E+03   .18267393E+03   .18193845E+03\n   .18112047E+03   .18022125E+03   .17924220E+03   .17818481E+03   .17705068E+03\n   .17584151E+03   .17455912E+03   .17320542E+03   .17178242E+03   .17029222E+03\n   .16873702E+03   .16711910E+03   .16544083E+03   .16370466E+03   .16191309E+03\n   .16006871E+03   .15817413E+03   .15623203E+03   .15424514E+03   .15221621E+03\n   .15014801E+03   .14804336E+03   .14590508E+03   .14373600E+03   .14153897E+03\n   .13931682E+03   .13707240E+03   .13480853E+03   .13252803E+03   .13023368E+03\n   .12792824E+03   .12561445E+03   .12329498E+03   .12097249E+03   .11864956E+03\n   .11632874E+03   .11401249E+03   .11170324E+03   .10940334E+03   .10711507E+03\n   .10484063E+03   .10258216E+03   .10034170E+03   .98121210E+02   .95922584E+02\n   .93747610E+02   .91597989E+02   .89475332E+02   .87381157E+02   .85316885E+02\n   .83283843E+02   .81283262E+02   .79316277E+02   .77383928E+02   .75487158E+02\n   .73626815E+02   .71803655E+02   .70018337E+02   .68271432E+02   .66563416E+02\n   .64894679E+02   .63265521E+02   .61676158E+02   .60126721E+02   .58617263E+02\n   .57147756E+02   .55718097E+02   .54328112E+02   .52977556E+02   .51666118E+02\n   .50393426E+02   .49159046E+02   .47962489E+02   .46803211E+02   .45680620E+02\n   .44594078E+02   .43542903E+02   .42526375E+02   .41543736E+02   .40594200E+02\n  
